vi "Prober_ChuckUpDown.vi"(8 "error in (no error)":errorcluster, 10 "Direction":enum16{"up", "down"}(ring), 11 "SemiProbe in":refnum<class "SemiProbe.lvclass">) -> (0 "error out":errorcluster, 2 "Chuck at CONTACT?":bool=TRUE, 3 "SemiProbe out":refnum<class "SemiProbe.lvclass">)   [LabVIEW 2019, in "SemiProbe.lvclass"]
uses:
  SemiProbe.lvclass
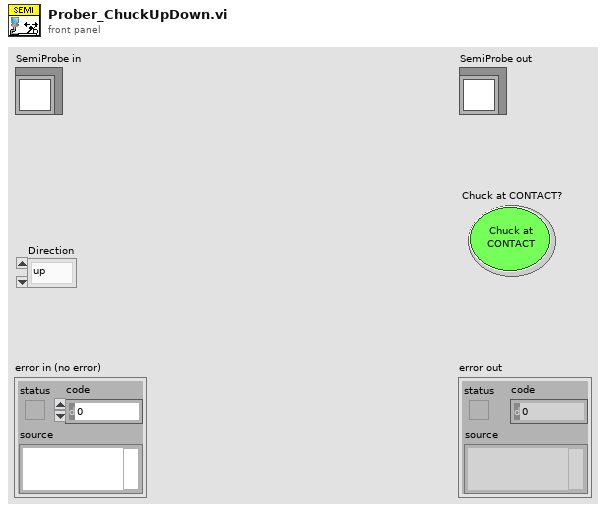
[diagram p1: front panel]
types:
  T1 = enum16{"Move To Load", "Move To Double Separation", "Move To Separation Distance", "Move To Contact", "Execute Contact Search", "Execute Arduino Contact Search"}
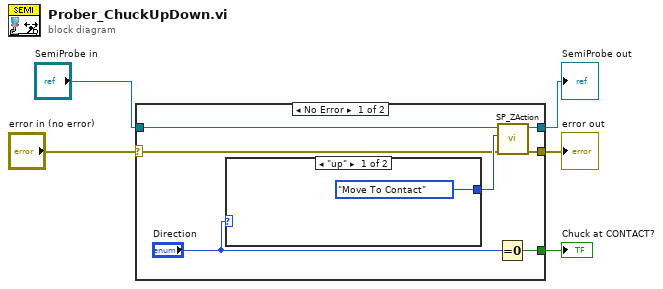
[diagram p0: block diagram]
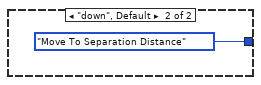
[diagram p2: hidden frame]
diagram:
  n1 = case shown="No Error" "error in (no error)" {
    selector: "error in (no error)" -> [w11 w15]
    tunnel: "SemiProbe in" -> [w10 w16]
    tunnel: [w7 w16] -> w3
    tunnel: [w6 w15] -> w2
    tunnel: [w8 _] -> w1
    frame No Error {
      n2 = case shown="\"up\"" "Direction" {
        tunnel: [T1."Move To Contact" ("Z Action") T1."Move To Separation Distance" ("Z Action")] -> w12
        frame "up" {
        }
        frame "down", Default {
        }
      }
      n3 = Equal To 0?(x="Direction") -> (x = 0?=w8:bool)
      n4 = call-dynamic "SP_ZAction.vi"("error in (no error)"=w11, "Z Action"=w12, "SemiProbe in"=w10) -> ("error out"=w6:errorcluster, "SemiProbe out"=w7:refnum<class "SemiProbe.lvclass">)  [unwired: 5 in, 2 out]
    }
    frame Error {
    }
  }
  "error out" <- w2
  "SemiProbe out" <- w3
  "Chuck at CONTACT?" <- w1
